vi "TempMonitor_SetLimits_SetTemp_CheckDigitalAlertSignal.vi"(0 "Serial Port to Use":refnum<visa-resource-name>="COM8", 1 "High Limit (C)":i32=60, 2 "Low Limit (C)":i32=-10, 3 "Sensor Temp (C)":dbl, 4 "Test Block Analog Output":tag="Dev1/ao0", 5 "Test Block Digital Alert Input":tag="Dev1/port0/line1") -> (14 "Pass":bool, 16 "Alert State":bool, 19 "error out":errorcluster)   [LabVIEW 2012]
uses:
  <vilib>/DAQmx/write.llb/DAQmx Write (Analog DBL 1Chan 1Samp).vi
  <vilib>/DAQmx/read.llb/DAQmx Read (Digital Bool 1Line 1Point).vi
  TempMonitor_Command_Enumerations.vi
  <vilib>/DAQmx/create/channels.llb/DAQmx Create Channel (AO-Voltage-Basic).vi
  <vilib>/DAQmx/miscellaneous.llb/DAQmx Fill In Error Info.vi
  <vilib>/DAQmx/create/channels.llb/DAQmx Create Channel (DI-Digital Input).vi
panel:
  out "Ack Received 2":bool
  out "Layer2 Payload 2":string
  out "A Packet Acked 2":bool
  out "Layer2 Payload 1":string
  out "Ack Received 1":bool
  out "A Packet Acked 1":bool
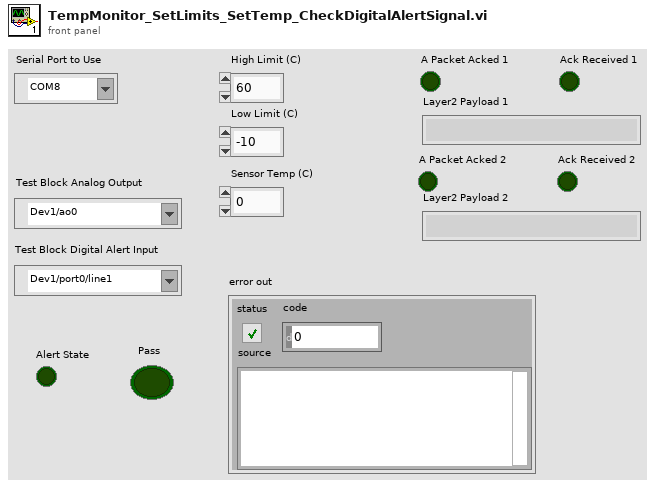
[diagram p1: front panel]
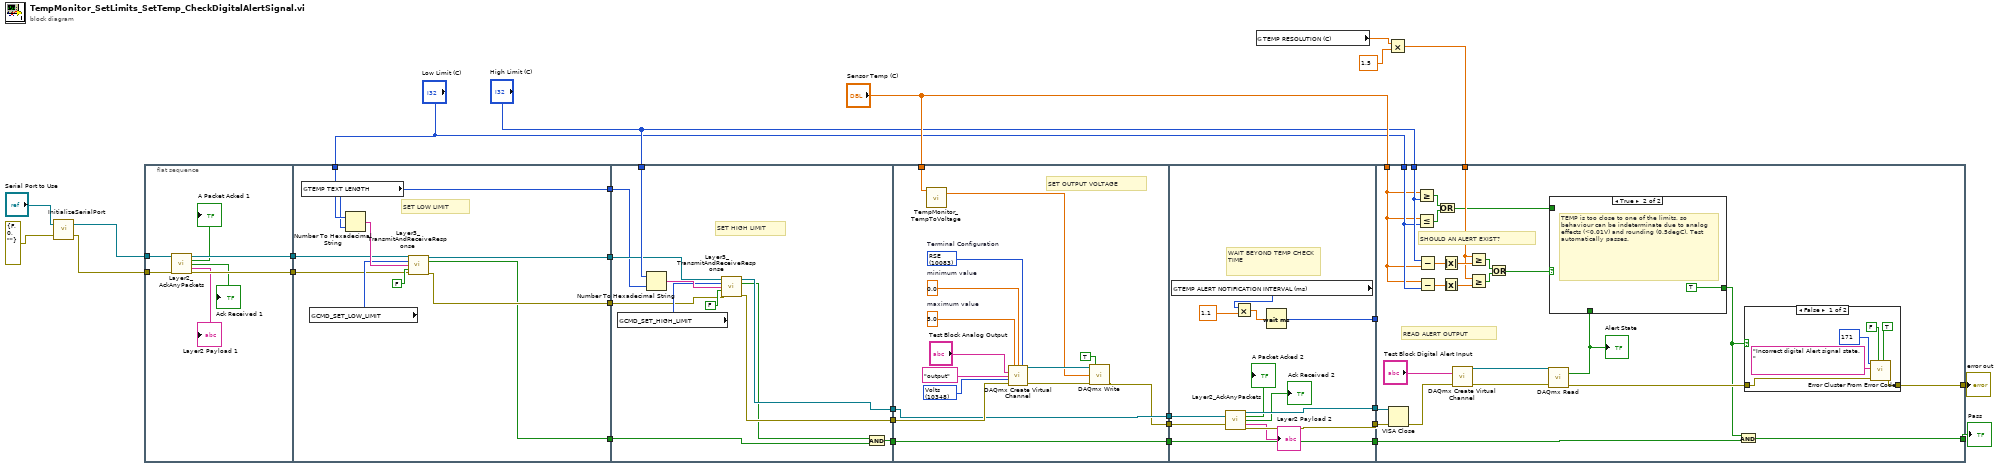
[diagram p0: block diagram]
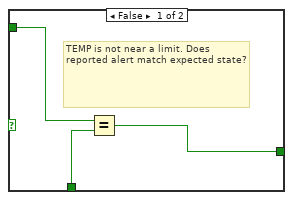
[diagram p3: hidden frame]
diagram:
  n1 = call "InitializeSerialPort.vi"("error in (no error)"=errorcluster {"status"=FALSE, "code"=0, "source"=""}, "Serial Port to Use"="Serial Port to Use") -> ("error out"=w6:errorcluster, "Configured Serial Port Identifier"=w5:refnum<visa-resource-name>)
  n2 = flat-sequence {
    tunnel: [w35] -> w8
    tunnel: [w34] -> w7
    tunnel: w6 -> [w33]
    tunnel: w5 -> [w32]
    tunnel: [w36] -> w28
    tunnel: "Low Limit (C)" -> [w42]
    tunnel: [w41] -> w15
    tunnel: [w40] -> w14
    tunnel: w8 -> [w39]
    tunnel: w7 -> [w38]
    tunnel: [w37] -> w1
    tunnel: w28 -> [w46]
    tunnel: [w48] -> w27
    tunnel: "High Limit (C)" -> [w54]
    tunnel: [w50] -> w18
    tunnel: w15 -> [w53]
    tunnel: w14 -> [w52]
    tunnel: [w51] -> w13
    tunnel: w1 -> [w49]
    tunnel: w27 -> [w61]
    tunnel: "Sensor Temp (C)" -> [w63]
    tunnel: [w61] -> w21
    tunnel: w18 -> [w60]
    tunnel: w13 -> [w59]
    tunnel: [w59] -> w12
    tunnel: [w58] -> w11
    tunnel: [w84] -> w26
    tunnel: [w83] -> w22
    tunnel: w21 -> [w83]
    tunnel: w12 -> [w82]
    tunnel: w11 -> [w81]
    tunnel: [w80] -> w10
    tunnel: [w79] -> w9
    tunnel: w26 -> [_]
    tunnel: "Sensor Temp (C)" -> [w97]
    tunnel: "High Limit (C)" -> [w103]
    tunnel: "Low Limit (C)" -> [w98]
    tunnel: [w89] -> w19
    tunnel: w22 -> [w105]
    tunnel: [w104] -> w20
    tunnel: w2 -> [w96]
    tunnel: w10 -> [w86]
    tunnel: w9 -> [w87]
    frame #0 {
      n3 = call "Layer2_AckAnyPackets.vi"("Serial Port to Use"=w32, "Error In"=w33) -> ("Serial Port to Use (out)"=w35:refnum<visa-resource-name>, "A Packet Acked"=→"A Packet Acked 1":bool, "Ack Received"=→"Ack Received 1":bool, "Layer2 Payload"=→"Layer2 Payload 1":string, "Error Out"=w34:errorcluster)  [unwired: 9 in]
    }
    frame #1 {
      # "SET LOW LIMIT"
      n4 = global read "TempMonitor_Command_Enumerations.vi" "TEMP TEXT LENGTH"() -> (w37:u8)
      n5 = global read "TempMonitor_Command_Enumerations.vi" "CMD_SET_LOW_LIMIT"() -> (w43:u16)
      n6 = Number To Hexadecimal String(1:w37, 2:w42) -> (0:w44:string)
      n7 = call "Layer3_TransmitAndReceiveResponse.vi"("Serial Port to Use"=w39, "CMD"=w43, "Message"=w44, "Expecting Response"=FALSE, "error in (no error)"=w38) -> ("Serial Port to Use (out)"=w41:refnum<visa-resource-name>, "Success"=w36:bool, "Error Out"=w40:errorcluster)  [unwired: 6 in, 2 out]
    }
    frame #2 {
      # "SET HIGH LIMIT"
      n8 = global read "TempMonitor_Command_Enumerations.vi" "CMD_SET_HIGH_LIMIT"() -> (w55:u16)
      n9 = Number To Hexadecimal String(1:w49, 2:w54) -> (0:w56:string)
      n10 = call "Layer3_TransmitAndReceiveResponse.vi"("Serial Port to Use"=w53, "CMD"=w55, "Message"=w56, "Expecting Response"=FALSE, "error in (no error)"=w52) -> ("Serial Port to Use (out)"=w51:refnum<visa-resource-name>, "Success"=w47:bool, "Error Out"=w50:errorcluster)  [unwired: 6 in, 2 out]
      n11 = And(x=w47, y=w46) -> (x .and. y?=w48:bool)
    }
    frame #3 {
      w64 = 10083 items=["Default"=-1, "RSE"=10083, "Differential"=10106, "Pseudodifferential"=12529]  # Terminal Configuration
      w66 = 5.0  # maximum value
      w65 = 0.0  # minimum value
      w67 = 10348 items=["Volts"=10348, "From Custom Scale"=10065] ("units")
      # "SET OUTPUT VOLTAGE"
      n12 = call "TempMonitor_TempToVoltage.vi"("Temp (C)"=w63) -> ("Output Voltage"=w62:dbl)  [unwired: 3 in, 1 out]
      n13 = call-poly <vilib>:"DAQmx Create Virtual Channel.vi"("maximum value"=w66, "minimum value"=w65, "output terminal configuration"=w64, "physical channels"="Test Block Analog Output", "name to assign"="output", "units"=w67, "error in"=w60) -> ("task out"=w72:refnum<k21>, "error out"=w71:errorcluster)  [unwired: 7 in]
      n14 = call-poly <vilib>:"DAQmx Write.vi"("task/channels in"=w72, "auto start"=TRUE, "data"=w62, "error in"=w71) -> ("error out"=w58:errorcluster)  [unwired: 9 in, 2 out]
    }
    frame #4 {
      # "WAIT BEYOND TEMP CHECK TIME"
      n15 = global read "TempMonitor_Command_Enumerations.vi" "TEMP ALERT NOTIFICATION INTERVAL (ms)"() -> (w75:u32)
      n16 = call "Layer2_AckAnyPackets.vi"("Serial Port to Use"=w82, "Error In"=w81) -> ("Serial Port to Use (out)"=w79:refnum<visa-resource-name>, "A Packet Acked"=→"A Packet Acked 2":bool, "Ack Received"=→"Ack Received 2":bool, "Layer2 Payload"=→"Layer2 Payload 2":string, "Error Out"=w80:errorcluster)  [unwired: 9 in]
      n17 = Multiply(x=w75, y=1.1) -> (x*y=w73:dbl)
      n18 = Wait (ms)(milliseconds to wait=w73) -> (millisecond timer value=w84:u32)
    }
    frame #5 {
      # "SHOULD AN ALERT EXIST?"
      # "READ ALERT OUTPUT"
      n19 = VISA Close(VISA resource name=w87, error in (no error)=w86) -> (error out=w85:errorcluster)
      n20 = Greater Or Equal?(x=w97, y=w103) -> (x >= y?=w110:bool)
      n21 = Less Or Equal?(x=w97, y=w98) -> (x <= y?=w109:bool)
      n22 = Subtract(x=w103, y=w97) -> (x-y=w102:dbl)
      n23 = Subtract(x=w97, y=w98) -> (x-y=w100:dbl)
      n24 = Or(x=w110, y=w109) -> (x .or. y?=w93:bool)
      n25 = Absolute Value(x=w102) -> (abs(x)=w101:dbl)
      n26 = Absolute Value(x=w100) -> (abs(x)=w99:dbl)
      n27 = call-poly <vilib>:"DAQmx Create Virtual Channel.vi"("lines"="Test Block Digital Alert Input", "error in"=w85) -> ("task out"=w108:refnum<k21>, "error out"=w107:errorcluster)  [unwired: 12 in]
      n28 = Greater Or Equal?(x=w96, y=w101) -> (x >= y?=w94:bool)
      n29 = Greater Or Equal?(x=w96, y=w99) -> (x >= y?=w95:bool)
      n30 = Or(x=w94, y=w95) -> (x .or. y?=w91:bool)
      n31 = call-poly <vilib>:"DAQmx Read.vi"("task/channels in"=w108, "error in"=w107) -> ("data"=w92:bool, "error out"=w90:errorcluster)  [unwired: 11 in, 1 out]
      "Alert State" <- w92
      n32 = case shown="True" w91 {
        tunnel: w93 -> [w120 _]
        tunnel: w92 -> [w119 _]
        tunnel: [w118 TRUE] -> w88
        frame False {
          # "TEMP is not near a limit. Does reported alert match expected state?"
          n33 = Equal?(x=w120, y=w119) -> (x = y?=w118:bool)
        }
        frame True {
          # "TEMP is too close to one of the limits, so behaviour can be indeterminate due to analog effects (<0.01V) and rounding (0.5degC). Test automatically passes."
        }
      }
      n34 = And(x=w88, y=w105) -> (x .and. y?=w104:bool)
      n35 = case shown="False" w88 {
        tunnel: w90 -> [w111 w117]
        tunnel: [w114 w117] -> w89
        frame False {
          n36 = call <vilib>:"Error Cluster From Error Code.vi"("is warning? (False)"=TRUE, "show call chain? (False)"=FALSE, "error in (no error)"=w111, "error message (\"\")"="Incorrect digital Alert signal state." ("source"), "error code (0)"=171 ("code")) -> ("error out"=w114:errorcluster)  [unwired: 4 in]
        }
        frame True {
        }
      }
    }
  }
  n37 = global read "TempMonitor_Command_Enumerations.vi" "TEMP RESOLUTION (C)"() -> (w4:dbl)
  n38 = Multiply(x=w4, y=1.5) -> (x*y=w2:dbl)
  "Pass" <- w20
  "error out" <- w19
